vi "00 DoubleCheck.vi"(8 "error in (no error)":errorcluster caption="错误输入（无错误）", 10 "服务端属性":cluster{"本机IP":string, "本机端口":u16}, 11 "TCPServerClass 输入":refnum<class "TCPServerClass.lvclass">) -> (0 "error out":errorcluster caption="错误输出", 2 "重复？":bool, 3 "TCPServerClass 输出":refnum<class "TCPServerClass.lvclass">)   [LabVIEW 2019, in "TCPServerClass.lvclass"]
uses:
  TCPServerClass.lvclass
  TCPServerClass.lvclass/TCPServerClass.ctl
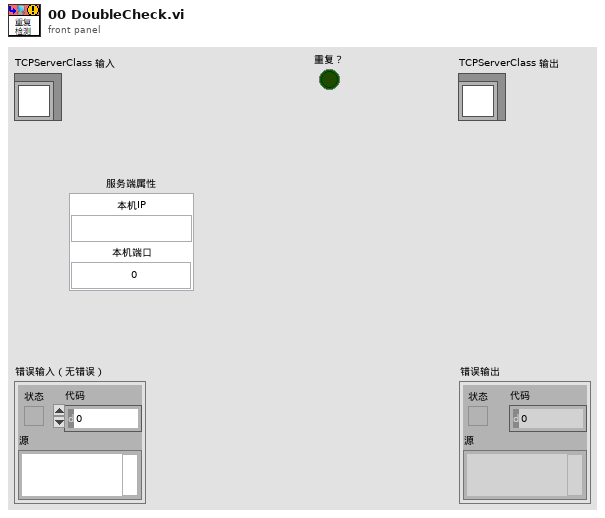
[diagram p1: front panel]
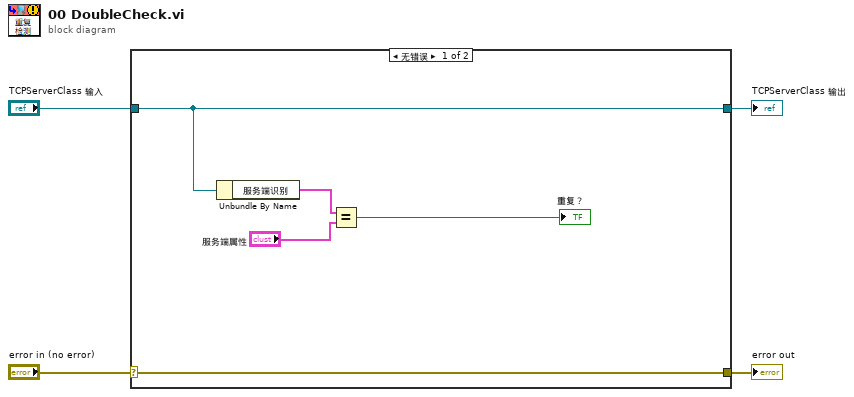
[diagram p0: block diagram]
diagram:
  n1 = case shown="无错误" "error in (no error)" {
    selector: "error in (no error)" -> [w9 w11]
    tunnel: [w9 w11] -> w3
    tunnel: [w8 w10] -> w1
    tunnel: "TCPServerClass 输入" -> [w8 w10]
    frame No Error {
      n2 = Unbundle By Name(w8) -> ("服务端识别"=w7:cluster{"本机IP":string, "本机端口":u16})
      n3 = Equal?(x=w7, y="服务端属性") -> (x = y?=→"重复？":bool)
    }
    frame Error {
    }
  }
  "error out" <- w3
  "TCPServerClass 输出" <- w1
